vi "set_electrodes (SubVI).vi"(8 "electrodes reference":refnum<vi>, 9 "electrodes error":errorcluster, 10 "electrodes task 2":refnum<k21>, 11 "Tot Electrode Arr":dbl[](array[numeric])) -> (0 "electrodes task error":errorcluster, 1 "DC volts arr":dbl[](array[numeric]), 2 "electrodes task":refnum<k21>, 3 "electrode arr":dbl[][](array[numeric]))   [LabVIEW 2014]
uses:
  <vilib>/measure/NI_MABase.lvlib
  <resource>/objmgr/daqmx.rc
panel:
  out "SampClk.Rate":dbl
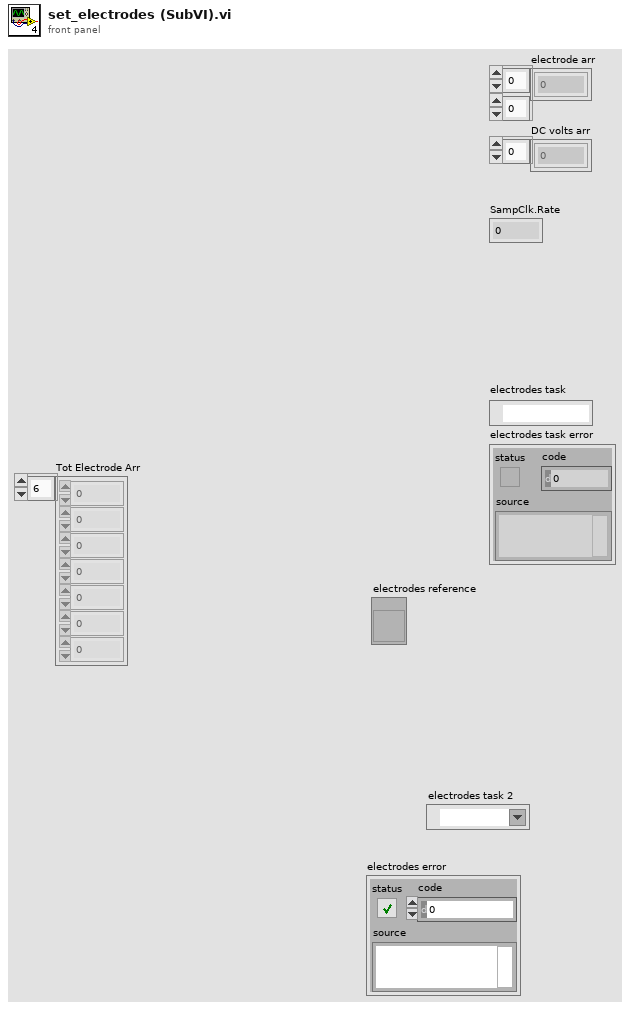
[diagram p1: front panel]
types:
  T1 = cluster{"DC volts (V):\n":dbl[], "Electrode to sweep:":i32, "start volt (V)":ext, "stop volt (V) ":ext, "# V Steps":i32, "start freq (Hz)":ext, "stop freq (Hz) ":ext, "# F steps":i32, "start DC (V)":ext, "stop DC (V)":ext, "# DC steps ":i32, "Digitize electrode\ndrives?":bool, "Sweep electrode?":bool, "Add 0.5*V DC \noffset for amp?":bool}
  T2 = enum16{"Sine Wave", "Triangle Wave", "Square Wave", "Sawtooth Wave"}
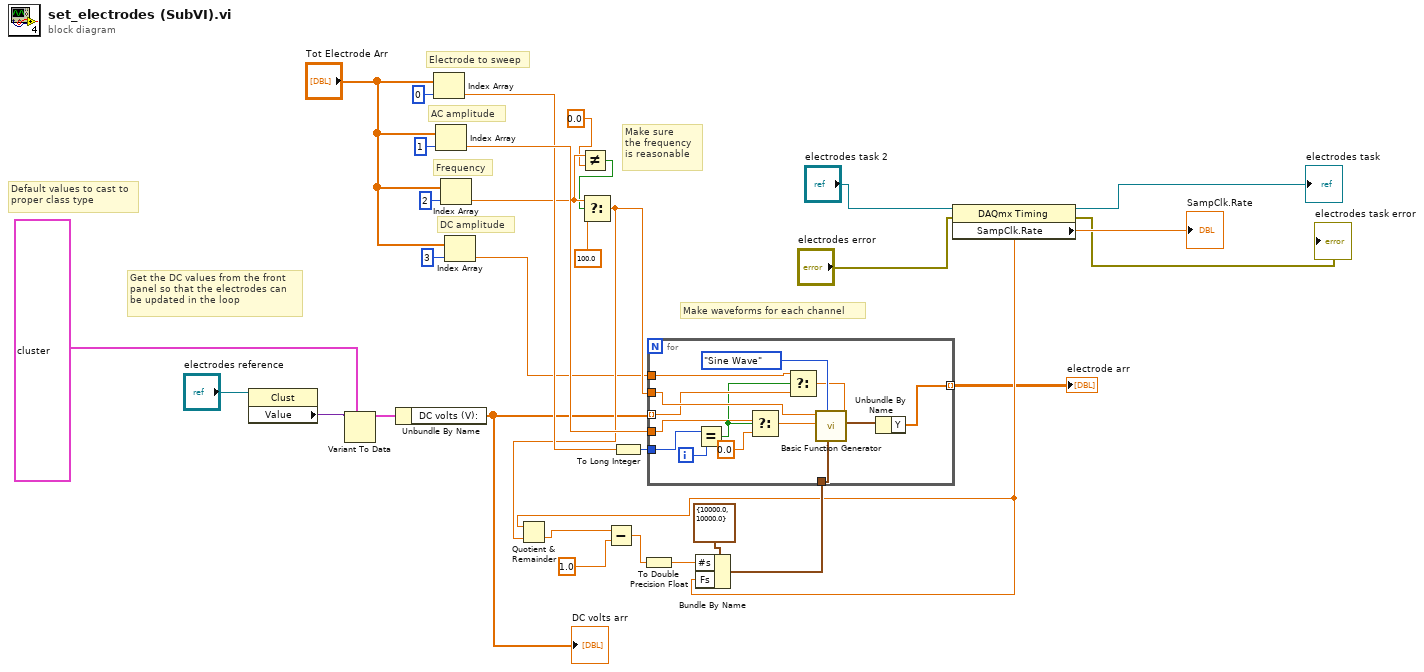
[diagram p0: block diagram]
diagram:
  # "Default values to cast to\nproper class type"
  # "Get the DC values from the front\npanel so that the electrodes can\nbe updated in the loop"
  # "Make sure\nthe frequency \nis reasonable"
  # "Make waveforms for each channel"
  # "DC amplitude"
  # "Frequency"
  # "AC amplitude"
  # "Electrode to sweep"
  n1 = property class="Clust"(reference="electrodes reference") -> ("Value"=w5:variant)  [unwired: 1 in, 2 out]
  n2 = Variant To Data(type=T1 {"DC volts (V):\n"=[0.0, 0.0, 0.0, 0.0, 0.0, 0.0, 0.0, 0.0], "Electrode to sweep:"=0, "start volt (V)"=1.0, "stop volt (V) "=1.0, "# V Steps"=1, "start freq (Hz)"=100.0, "stop freq (Hz) "=100.0, "# F steps"=1, "start DC (V)"=0.0, "stop DC (V)"=0.0, "# DC steps "=1, "Digitize electrode\ndrives?"=TRUE, "Sweep electrode?"=TRUE, "Add 0.5*V DC \noffset for amp?"=FALSE} ("Electrode settings:"), Variant=w5) -> (data=w4:T1)  [unwired: 1 in, 1 out]
  n3 = Unbundle By Name(w4) -> ("DC volts (V):"=w3:dbl[])
  "DC volts arr" <- w3
  n4 = Index Array(array="Tot Electrode Arr", index=0) -> (element=w21:dbl)
  n5 = Index Array(array="Tot Electrode Arr", index=1) -> (element=w22:dbl)
  n6 = Index Array(array="Tot Electrode Arr", index=2) -> (element=w15:dbl)
  n7 = Index Array(array="Tot Electrode Arr", index=3) -> (element=w2:dbl)
  n8 = Not Equal?(x=w15, y=0.0) -> (x != y?=w13:bool)
  n9 = Select(t=w15, s=w13, f=100.0) -> (s? t:f=w17:dbl)
  n10 = To Long Integer(number=w21) -> (32bit integer=w20:i32)
  n11 = property class="DAQmx Timing"(reference="electrodes task 2", error in="electrodes error") -> (reference out=→"electrodes task":refnum<k21>, error out=→"electrodes task error":errorcluster, "SampClk.Rate"=w10:dbl)
  "SampClk.Rate" <- w10
  n12 = Quotient & Remainder(x=w10, y=w17) -> (floor(x/y)=w25:dbl)  [unwired: 1 out]
  n13 = Subtract(x=w25, y=1.0) -> (x-y=w23:dbl)
  n14 = To Double Precision Float(number=w23) -> (double precision float=w26:dbl)
  n15 = Bundle By Name(cluster=cluster{"Fs":dbl, "#s":dbl} {"Fs"=10000.0, "#s"=10000.0} ("sampling info"), "#s"=w26, "Fs"=w10) -> (w19:cluster{"Fs":dbl, "#s":dbl})
  n16 = for {
    tunnel: w3 -> [w35] mode=indexing
    tunnel: w17 -> [w44]
    tunnel: w22 -> [w41]
    tunnel: w20 -> [w39]
    tunnel: w19 -> [w38]
    tunnel: [w36] -> w9 mode=indexing
    tunnel: w2 -> [w33]
    i -> [w40]
    n17 = Equal?(x=w39, y=w40) -> (x = y?=w32:bool)
    n18 = Select(t=w41, s=w32, f=0.0) -> (s? t:f=w43:dbl)
    n19 = Select(t=w33, s=w32, f=w35) -> (s? t:f=w34:dbl)
    n20 = call <vilib>:"Basic Function Generator.vi"("offset"=w34, "sampling info"=w38, "signal type"=T2."Sine Wave", "amplitude"=w43, "frequency"=w44) -> ("signal out"=w37:waveform(dbl))  [unwired: 4 in, 2 out]
    n21 = Unbundle By Name(w37) -> ("Y"=w36:dbl[])
  }
  "electrode arr" <- w9
